vi "数据写入database.vi"(9 "data":variant, 10 "columns":string[](array[string]), 11 "table":string) -> (1 "error out":errorcluster)   [LabVIEW 2016, in "斯坦道CODMn.lvlib"]
uses:
  <vilib>/Utility/sysdir.llb/System Directory Type.ctl
  <vilib>/Utility/error.llb/DialogType.ctl
  <vilib>/addons/database/Auxilliary.llb/DB Tools Transaction.ctl
  <vilib>/addons/database/Auxilliary.llb/DB Tools Isolation Level.ctl
  <vilib>/addons/database/Auxilliary.llb/DB Tools Column Info.ctl
  <vilib>/addons/database/Auxilliary.llb/DB Tools DataTypes.ctl
  <vilib>/addons/database/Connection.llb/DB Tools Open Connec (String).vi
  <vilib>/addons/database/Connection.llb/Conn Execute.vi
  <vilib>/addons/database/Recordset.llb/Rec Destroy - Connection.vi
  <vilib>/addons/database/Recordset.llb/Rec Fetch Recordset Data (R).vi
  <vilib>/addons/database/Connection.llb/Conn Transaction.vi
  <vilib>/addons/database/NI_Database_API.lvlib
  WxMessage/wxpusher.lvlib
panel:
  out "修正数据":T1
  out "数据":T1
  out "为空？":bool
  in  "error in (no error)":errorcluster
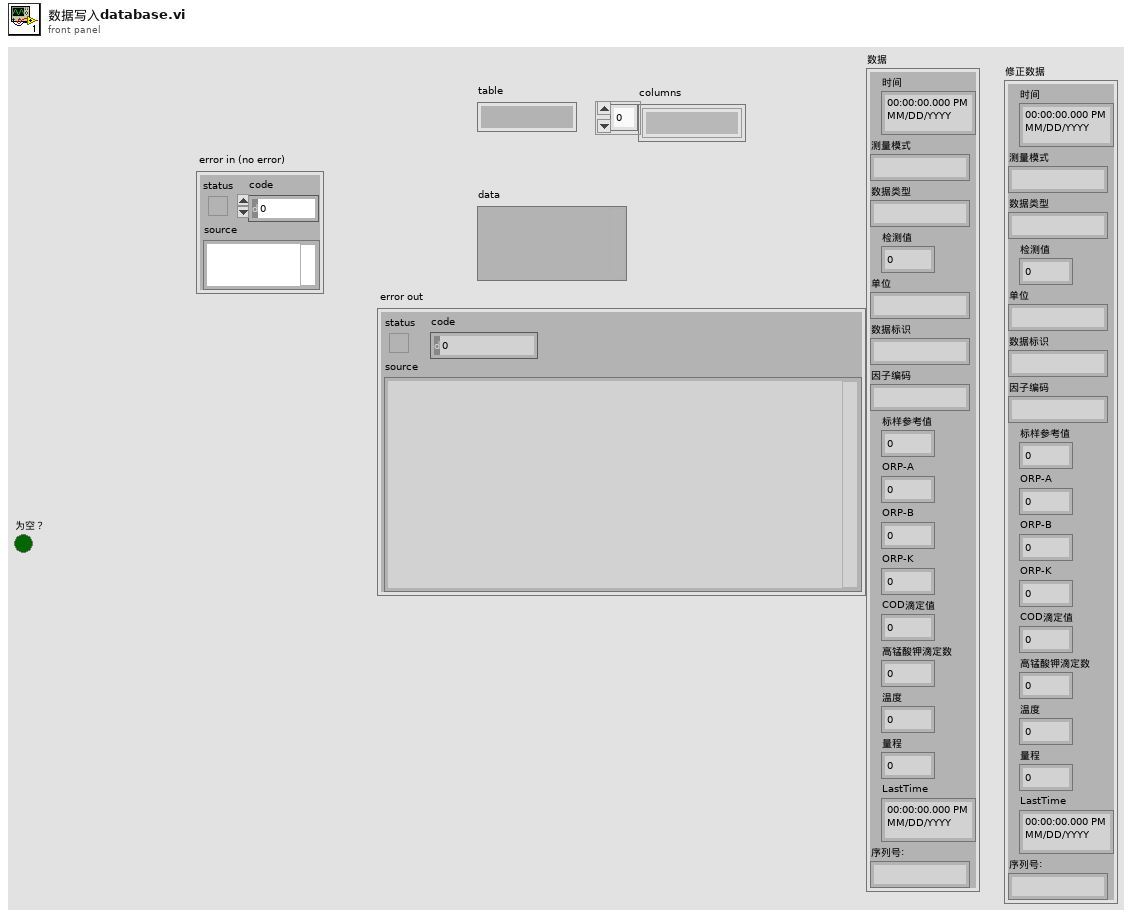
[diagram p1: front panel]
types:
  T1 = cluster{"时间":timestamp, "测量模式":string, "数据类型":string, "检测值":sgl, "单位":string, "数据标识":string, "因子编码":string, "标样参考值":sgl, "ORP-A":sgl, "ORP-B":sgl, "ORP-K":sgl, "COD滴定值":sgl, "高锰酸钾滴定数":sgl, "温度":sgl, "量程":sgl, "LastTime":timestamp, "序列号:":string}
  T2 = typedef "DialogType.ctl" = u16
  T3 = typedef "System Directory Type.ctl" = i32
  T4 = typedef "NI_Database_API.lvlib/Conn ObjectReference.ctl" = refnum<k1>
  T5 = typedef "NI_Database_API.lvlib/Rec ObjectReference.ctl" = refnum<k1>
  T6 = typedef "NI_Database_API.lvlib/DB Tools Transaction.ctl" = enum16{"begin", "commit", "rollback"}
  T7 = typedef "NI_Database_API.lvlib/DB Tools Isolation Level.ctl" = enum16{"chaos", "read uncommitted", "read committed", "repeatable read", "serializable"}
  T8 = typedef "NI_Database_API.lvlib/DB Tools Column Info.ctl" = cluster{"column name":string, "data type":T9, "size":i32, "allow null?":bool}
  T9 = typedef "NI_Database_API.lvlib/DB Tools DataTypes.ctl" = enum16{"String", "Long (I32)", "Single (SGL)", "Double (DBL)", "Date/Time", "Binary"}
  T10 = cluster{"时间标识":timestamp, "设备":string, "日志信息":string}
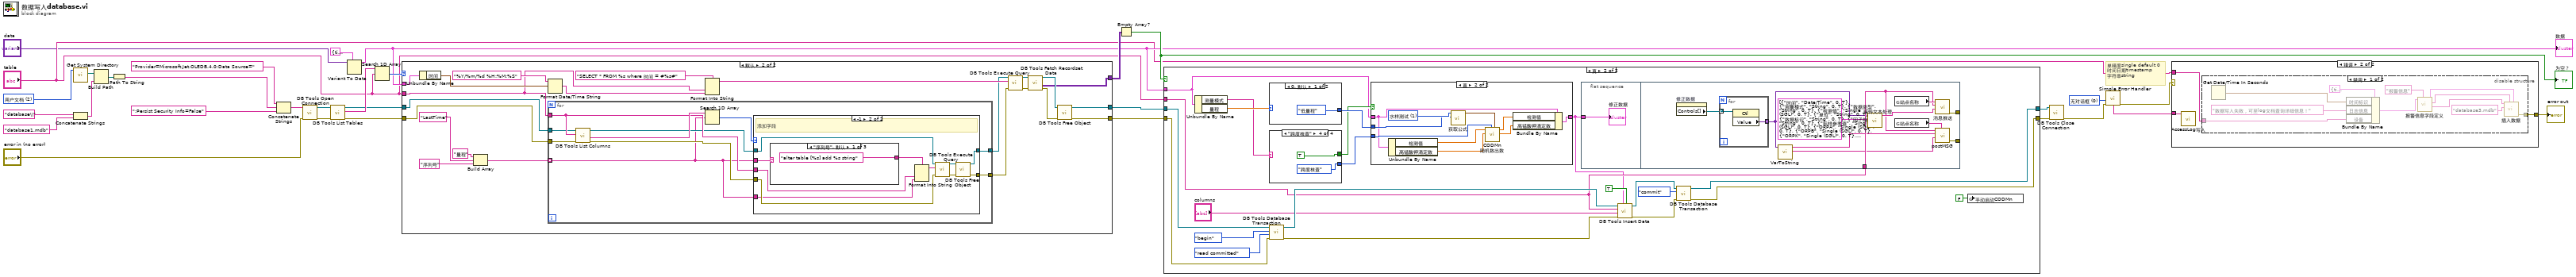
[diagram p0: block diagram]
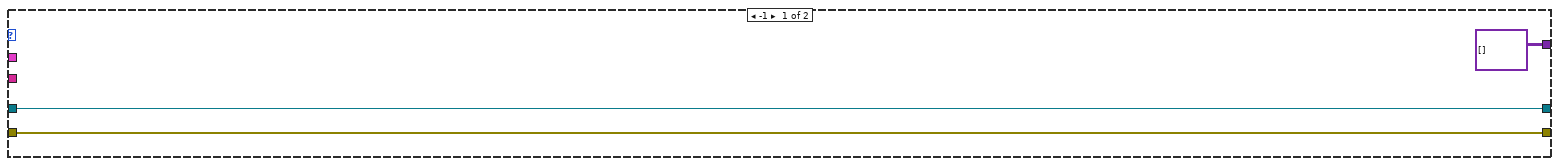
[diagram p4: hidden frame]
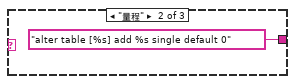
[diagram p6: hidden frame]
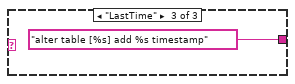
[diagram p7: hidden frame]
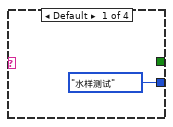
[diagram p10: hidden frame]
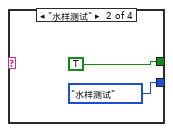
[diagram p11: hidden frame]
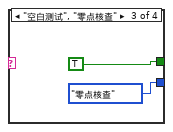
[diagram p12: hidden frame]
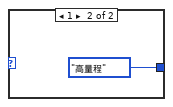
[diagram p13: hidden frame]
diagram:
  w8 = T2 0 items=["无对话框", "确定信息", "继续或停止信息", "确定信息＋警告", "继续/停止+警告"] ("type of dialog (OK msg:1)")
  w32 = T3 2 items=["用户目录"=0, "用户桌面"=1, "用户文档"=2, "用户应用程序数据"=3, "用户设置"=4, "用户临时目录"=5, "公共文档"=6, "公共应用程序数据"=7, "公共设置"=8, "公共缓存"=13, "系统核心库"=9, "系统安装库"=10, "应用程序文件"=11, "启动盘根目录"=12] ("system directory type")
  # "单精度single default 0\n时间日期timestamp\n字符串string"
  n1 = call <vilib>:"Get System Directory.vi"("system directory type"=w32) -> ("system directory"=w30:path)  [unwired: 10 in]
  n2 = Concatenate Strings("database\\" ("condition"), "database1.mdb" ("字符串")) -> (w24:string)
  n3 = Build Path(base path=w30, name or relative path=w24) -> (appended path=w29:path)
  n4 = Path To String(path=w29) -> (string=w28:string)
  n5 = Concatenate Strings("Provider=Microsoft.Jet.OLEDB.4.0;Data Source=" ("condition"), w28, ";Persist Security Info=False" ("condition")) -> (w26:string)
  n6 = call-poly <vilib>:"DB Tools Open Connection.vi"("error in (no error)"="error in (no error)", "connection information"=w26) -> ("error out"=w22:errorcluster, "connection reference"=w23:T4)  [unwired: 6 in]
  n7 = call <vilib>:"DB Tools List Tables.vi"("error in (no error)"=w22, "connection reference"=w23) -> ("error out"=w16:errorcluster, "tables"=w21:string[], "connection reference out"=w17:T4)  [unwired: 3 in]
  n8 = Variant To Data(type=T1 {"时间"=timestamp(0 s since 1904-01-01), "测量模式"="", "数据类型"="", "检测值"=0.0, "单位"="", "数据标识"="", "因子编码"="", "标样参考值"=0.0, "ORP-A"=0.0, "ORP-B"=0.0, "ORP-K"=0.0, "COD滴定值"=0.0, "高锰酸钾滴定数"=0.0, "温度"=0.0, "量程"=0.0, "LastTime"=timestamp(0 s since 1904-01-01), "序列号:"=""} ("data"), Variant="data") -> (data=w9:T1)  [unwired: 1 in, 1 out]
  "数据" <- w9
  n9 = Search 1D Array(1D array=w21, element="table") -> (index of element=w18:i32)  [unwired: 1 in]
  n10 = case shown="默认" w18 {
    tunnel: [variant[][] [] ("recordset data") w46] -> w15
    tunnel: [w35 w53] -> w14
    tunnel: [w34 w52] -> w13
    tunnel: w17 -> [w35 w40]
    tunnel: w16 -> [w34 w39]
    tunnel: "table" -> [_ w38]
    tunnel: w9 -> [_ w47]
    frame -1 {
    }
    frame Default {
      n11 = Unbundle By Name(w47) -> ("时间"=w50:timestamp)
      n12 = Build Array("量程" ("元素"), "LastTime" ("元素"), "序列号" ("元素")) -> (w44:string[])
      n13 = Format Date/Time String(time format string (%c)="%Y/%m/%d %H:%M:%S" ("时间格式字符串(%c)"), seconds (now)=w50) -> (date/time string=w48:string)  [unwired: 1 in]
      n14 = for {
        tunnel: w38 -> [w65]
        tunnel: w44 -> [w62] mode=indexing
        tunnel: [w61] -> w37
        tunnel: [w60] -> w36
        tunnel: w40 -> [w59]
        tunnel: w39 -> [w58]
        n15 = call <vilib>:"DB Tools List Columns.vi"("error in (no error)"=w58, "table"=w65, "connection reference"=w59) -> ("error out"=w63:errorcluster, "columns"=w67:string[], "connection reference out"=w64:T4)  [unwired: 1 in, 1 out]
        n16 = Search 1D Array(1D array=w67, element=w62) -> (index of element=w66:i32)  [unwired: 1 in]
        n17 = case shown="-1" w66 {
          tunnel: w64 -> [w69 w78]
          tunnel: w63 -> [w68 w77]
          tunnel: w62 -> [_ w76]
          tunnel: [w69 w74] -> w61
          tunnel: [w68 w73] -> w60
          tunnel: w65 -> [_ w72]
          tunnel: w62 -> [_ w71]
          frame 0, Default {
          }
          frame -1 {
            # "添加字段"
            n18 = case shown="\"序列号\", 默认" w71 {
              tunnel: ["alter table [%s] add %s string" "alter table [%s] add %s single default 0" "alter table [%s] add %s timestamp"] -> w70
              frame "序列号", Default {
              }
              frame "量程" {
              }
              frame "LastTime" {
              }
            }
            n19 = Format Into String(format string=w70, w72, w76) -> (resulting string=w75:string)  [unwired: 2 in, 1 out]
            n20 = call-poly <vilib>:"DB Tools Execute Query.vi"("error in (no error)"=w77, "SQL query"=w75, "connection reference"=w78) -> ("error out"=w79:errorcluster, "recordset reference"=w80:T5)  [unwired: 5 in]
            n21 = call-poly <vilib>:"DB Tools Free Object.vi"("error in (no error)"=w79, "recordset reference"=w80) -> ("error out"=w73:errorcluster, "connection reference"=w74:T4)  [unwired: 8 in]
          }
        }
      }
      n22 = Format Into String(format string="SELECT * FROM %s where 时间 = #%s#" ("格式字符串"), w38, w48) -> (resulting string=w51:string)  [unwired: 2 in, 1 out]
      n23 = call-poly <vilib>:"DB Tools Execute Query.vi"("error in (no error)"=w36, "SQL query"=w51, "connection reference"=w37) -> ("error out"=w54:errorcluster, "recordset reference"=w57:T5)  [unwired: 5 in]
      n24 = call-poly <vilib>:"DB Tools Fetch Recordset Data.vi"("error in (no error)"=w54, "recordset reference"=w57) -> ("error out"=w55:errorcluster, "recordset data"=w46:variant[][], "recordset reference out"=w56:T5)  [unwired: 3 in]
      n25 = call-poly <vilib>:"DB Tools Free Object.vi"("error in (no error)"=w55, "recordset reference"=w56) -> ("error out"=w52:errorcluster, "connection reference"=w53:T4)  [unwired: 8 in]
    }
  }
  n26 = Empty Array?(array=w15) -> (empty?=w10:bool)
  "为空？" <- w10
  n27 = case shown="真" w10 {
    tunnel: "table" -> [_ w93]
    tunnel: w9 -> [_ w87]
    tunnel: w13 -> [w84 w101]
    tunnel: w14 -> [w85 w102]
    tunnel: [w85 w96] -> w20
    tunnel: [w84 w95] -> w19
    frame False {
    }
    frame True {
      n28 = Unbundle By Name(w87) -> ("测量模式"=w90:string, "量程"=w92:sgl)
      n29 = case shown="0, 默认" w92 {
        tunnel: [enum16{"低量程", "高量程", "0-2量程"}."低量程" ("量程选择") enum16{"低量程", "高量程", "0-2量程"}."高量程" ("量程选择")] -> w91
        frame 0, Default {
        }
        frame 1 {
        }
      }
      n30 = case shown="\"跨度核查\"" w90 {
        tunnel: [enum16{"水样测试", "零点核查", "跨度核查"}."水样测试" ("测试模式") enum16{"水样测试", "零点核查", "跨度核查"}."水样测试" ("测试模式") enum16{"水样测试", "零点核查", "跨度核查"}."零点核查" ("测试模式") enum16{"水样测试", "零点核查", "跨度核查"}."跨度核查" ("测试模式")] -> w89
        tunnel: [_ TRUE TRUE TRUE] -> w88
        frame Default {
        }
        frame "水样测试" {
        }
        frame "空白测试", "零点核查" {
        }
        frame "跨度核查" {
        }
      }
      n31 = call-poly <vilib>:"DB Tools Database Transaction.vi"("error in (no error)"=w101, "isolation level (chaos)"=DB_Tools_Isolation_Level."read committed", "operation (begin)"=DB_Tools_Transaction."begin", "connection reference"=w102) -> ("error out"=w99:errorcluster, "connection reference out"=w100:T4)  [unwired: 2 in]
      n32 = case shown="真" w88 {
        tunnel: w91 -> [_ w116]
        tunnel: w89 -> [_ w115]
        tunnel: w87 -> [w108 w112]
        tunnel: [w108 w109] -> w86
        frame False {
        }
        frame True {
          w118 = u16 1 items=["水样测试"=1, "标样核查"=2, "零点核查"=3, "跨度核查"=4, "空白测试"=5, "平行样"=6, "加标回收"=7] ("测量模式(公式)")
          n33 = Unbundle By Name(w112) -> ("检测值"=w114:sgl, "高锰酸钾滴定数"=w113:sgl)
          n34 = call "获取公式.vi"("量程选择"=w116, "测量模式(公式)"=w118) -> ("方程系数"=w117:cluster{"K":dbl, "b":dbl, "X^2":dbl})  [unwired: 9 in]
          n35 = call "CODMn 随机数出数.vi"("公式"=w117, "测试模式"=w115, "信号值原始值"=w113, "原始值"=w114) -> ("信号值"=w110:dbl, "取值输出"=w111:dbl)  [unwired: 4 in]
          n36 = Bundle By Name(cluster=w112, "检测值"=w111, "高锰酸钾滴定数"=w110) -> (w109:T1)
        }
      }
      n37 = flat-sequence {
        tunnel: w86 -> [w128]
        tunnel: [w135] -> _
        tunnel: w93 -> [w133]
        tunnel: [w132] -> _
        frame #0 {
          "修正数据" <- w128
        }
        frame #1 {
          n38 = property on="修正数据" class="Clust (严格)"() -> ("Controls[]"=w137:refnum<vi>[])  [unwired: 2 in, 2 out]
          n39 = for {
            tunnel: w137 -> [w141] mode=indexing
            tunnel: [w140] -> w131 mode=indexing
            n40 = property class="Ctl"(reference=w141) -> ("Value"=w140:variant)  [unwired: 1 in, 2 out]
          }
          n41 = call "VarToString.vi"("数组"=w131) -> ("data"=w129:string[], "columns"=w130:string[])  [unwired: 9 in]
          n42 = call "簇转文本处理.vi"("column information"=T8[] [{"column name"="时间", "data type"=enum."Date/Time", "size"=0, "allow null?"=TRUE}, {"column name"="测量模式", "data type"=enum."String", "size"=0, "allow null?"=TRUE}, {"column name"="数据类型", "data type"=enum."String", "size"=0, "allow null?"=TRUE}, {"column name"="检测值", "data type"=enum."Single (SGL)", "size"=0, "allow null?"=TRUE}, {"column name"="单位", "data type"=enum."String", "size"=0, "allow null?"=TRUE}, {"column name"="数据标识", "data type"=enum."String", "size"=0, "allow null?"=TRUE}, {"column name"="因子编码", "data type"=enum."String", "size"=0, "allow null?"=TRUE}, {"column name"="标样参考值", "data type"=enum."Single (SGL)", "size"=0, "allow null?"=TRUE}, {"column name"="ORPA", "data type"=enum."Single (SGL)", "size"=0, "allow null?"=TRUE}, {"column name"="ORPB", "data type"=enum."Single (SGL)", "size"=0, "allow null?"=TRUE}, {"column name"="ORPK", "data type"=enum."Single (SGL)", "size"=0, "allow null?"=TRUE}, {"column name"="COD滴定值", "data type"=enum."Single (SGL)", "size"=0, "allow null?"=TRUE}, {"column name"="高锰酸盐滴定数", "data type"=enum."Single (SGL)", "size"=0, "allow null?"=TRUE}, {"column name"="温度", "data type"=enum."Single (SGL)", "size"=0, "allow null?"=TRUE}, {"column name"="湿度", "data type"=enum."Single (SGL)", "size"=0, "allow null?"=TRUE}, {"column name"="量程", "data type"=enum."Single (SGL)", "size"=0, "allow null?"=TRUE}, {"column name"="LastTime", "data type"=enum."Date/Time", "size"=0, "allow null?"=TRUE}, {"column name"="SN", "data type"=enum."String", "size"=0, "allow null?"=TRUE}], "data"=w131) -> ("output"=w139:string)  [unwired: 9 in]
          n43 = global read "系统设置全局变量.vi" "站点名称"() -> (w138:string)
          n44 = global read "系统设置全局变量.vi" "站点名称"() -> (w134:string)
          n45 = call "消息推送.vi"("分析"=w139, "内容"=w133, "站点"=w138) -> ("error out"=w135:errorcluster)  [unwired: 8 in]
          n46 = call "postMSG.vi"("station"=w134, "data"=w129, "columns"=w130, "table"=w133) -> ("error out"=w132:errorcluster)  [unwired: 7 in]
        }
      }
      n47 = call <vilib>:"DB Tools Insert Data.vi"("create table? (F)"=TRUE, "data"=w86, "error in (no error)"=w99, "columns"="columns", "table"=w93, "connection reference"=w100) -> ("error out"=w97:errorcluster, "connection reference out"=w98:T4)  [unwired: 4 in]
      n48 = call-poly <vilib>:"DB Tools Database Transaction.vi"("error in (no error)"=w97, "operation (begin)"=DB_Tools_Transaction."commit", "connection reference"=w98) -> ("error out"=w95:errorcluster, "connection reference out"=w96:T4)  [unwired: 3 in]
      n49 = global write "CODMN外部API.vi" "手动启动CODMn"(FALSE ("手动启动CODMn")) -> ()
    }
  }
  n50 = call <vilib>:"DB Tools Close Connection.vi"("error in (no error)"=w19, "connection reference"=w20) -> ("error out"=w6:errorcluster)  [unwired: 5 in]
  n51 = call <vilib>:"Simple Error Handler.vi"("type of dialog (OK msg:1)"=w8, "error in (no error)"=w6) -> ("error out"=w7:errorcluster, "message"=w3:string)  [unwired: 3 in, 3 out]
  n52 = case shown="错误" w7 {
    tunnel: "table" -> [_ w144]
    tunnel: [_ w143] -> w4
    tunnel: w3 -> [_ w142]
    frame No Error {
    }
    frame Error {
      n53 = call "AccessLog写入.vi"("Log"=w142) -> ()  [unwired: 11 in]
      n54 = disable-structure shown="禁用" {
        disable-tunnel: w144 -> [w153 _]
        disable-tunnel: [w146 _] -> w143
        frame Disabled {
          n55 = Get Date/Time In Seconds() -> (seconds since 1Jan1904=w154:timestamp)
          n56 = Bundle By Name(cluster=T10 {"时间标识"=timestamp(0 s since 1904-01-01), "设备"="氨氮", "日志信息"=""} ("data in"), "时间标识"=w154, "日志信息"="数据写入失败，可至log文档查询详细信息！" ("table输入"), "设备"=w153) -> (w147:T10)
          n57 = call "报警信息字段定义.vi"("table输入"="报警信息", "data in"=w147) -> ("table输出"=w150:string, "columns"=w151:string[], "data out"=w152:T10)  [unwired: 7 in]
          n58 = call "插入数据.vi"("data"=w152, "columns"=w151, "database"="database3.mdb", "table"=w150) -> ("error out"=w146:errorcluster)  [unwired: 7 in]
        }
        frame Enabled {
        }
      }
    }
  }
  "error out" <- w4
